vi "test_point.vi"() -> ()   [LabVIEW 2017]
panel:
  in  "stop":bool
  in  "P cluster":T1
  in  "T cluster":T2
  in  "Draw Points":bool
  in  "Cycle":string(combo)
  out "Table":string[][](table)
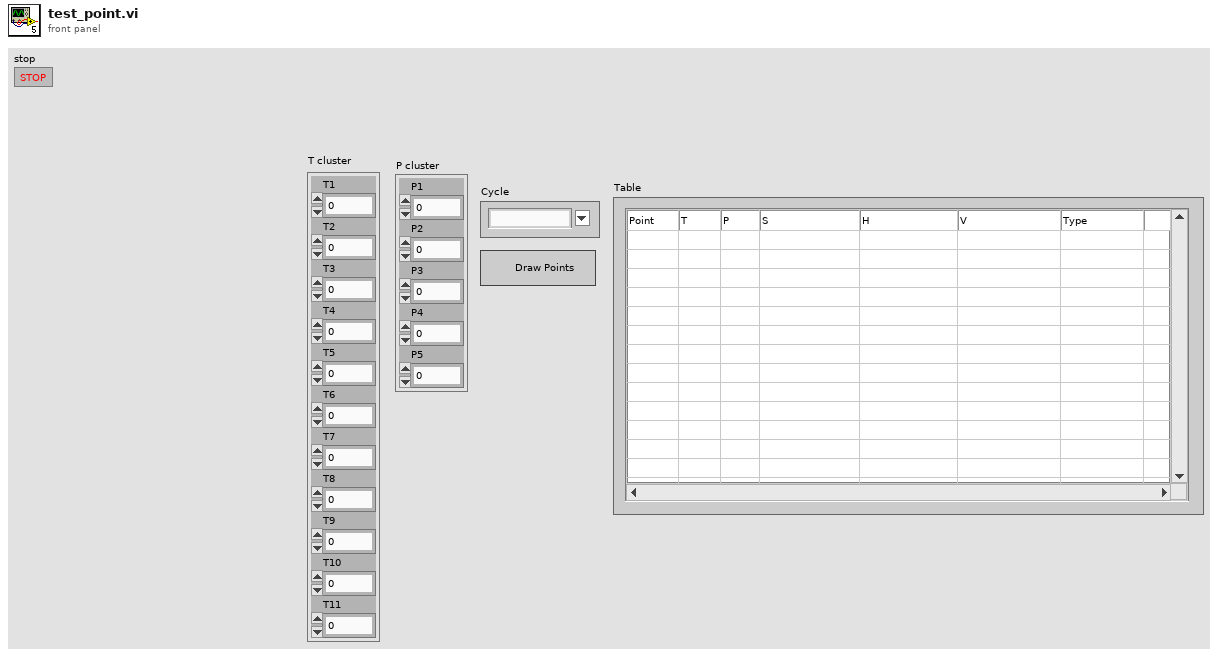
[diagram p1: front panel]
types:
  T1 = cluster{"P1":dbl, "P2":dbl, "P3":dbl, "P4":dbl, "P5":dbl}
  T2 = cluster{"T1":dbl, "T2":dbl, "T3":dbl, "T4":dbl, "T5":dbl, "T6":dbl, "T7":dbl, "T8":dbl, "T9":dbl, "T10":dbl, "T11":dbl}
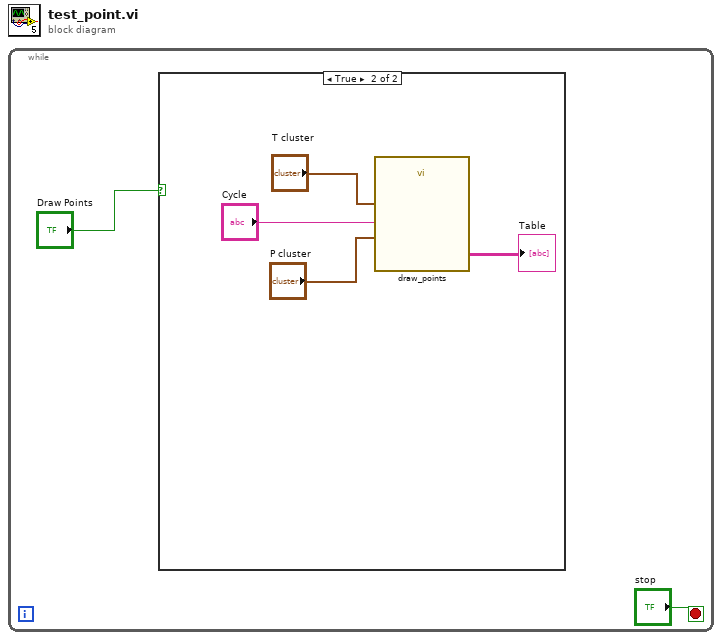
[diagram p0: block diagram]
diagram:
  n1 = while {
    stop <- "stop" stop-if-true
    n2 = case shown="True" "Draw Points" {
      frame False {
      }
      frame True {
        n3 = call "draw_points.vi"("Cycle"="Cycle", "T cluster"="T cluster", "P cluster"="P cluster") -> ("Table"=→"Table":string[][])  [unwired: 8 in]
      }
    }
  }
